vi "Sleep.vi"(8 "error in (no error)":errorcluster, 11 "ISleepableBaby in":refnum<class "ISleepableBaby.lvclass">) -> (0 "error out":errorcluster, 3 "ISleepableBaby out":refnum<class "ISleepableBaby.lvclass">)   [LabVIEW 2009, in "ISleepableBaby.lvclass"]
doc: "Cuddle with baby until she goes to sleep."
uses:
  ISleepableBaby.lvclass
  Baby.lvclass
  Source/IUnknown Class/IUnknown.lvclass
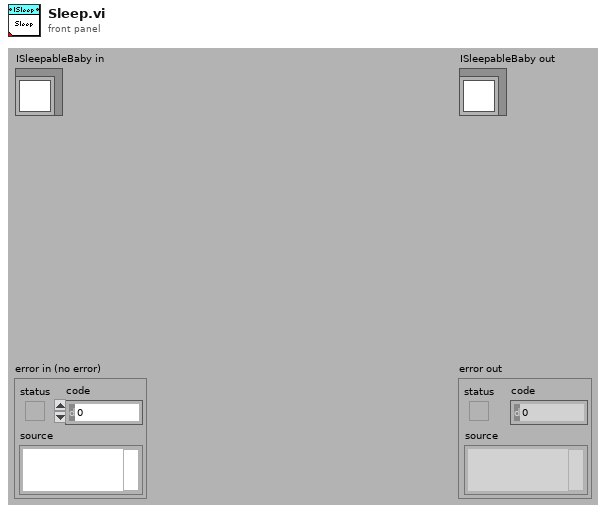
[diagram p1: front panel]
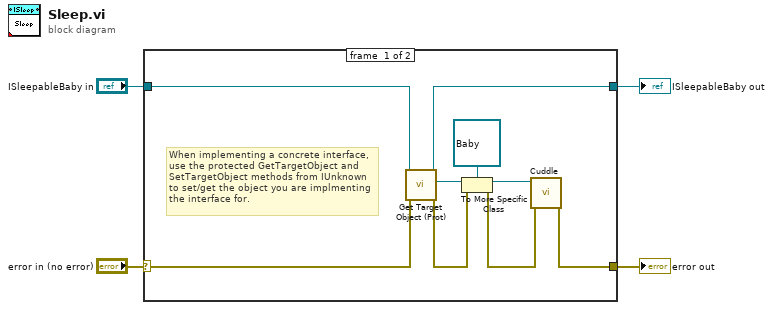
[diagram p0: block diagram]
diagram:
  n1 = case shown="No Error" "error in (no error)" {
    selector: "error in (no error)" -> [w5 w14]
    tunnel: "ISleepableBaby in" -> [w13 w15]
    tunnel: [w12 w15] -> w3
    tunnel: [w6 w14] -> w2
    frame #0 {
      # "When implementing a concrete interface,\nuse the protected GetTargetObject and SetTargetObject methods from IUnknown to set/get the object you are implmenting the interface for."
      n2 = call "Get Target Object (Prot).vi"("error in (no error)"=w5, "IUnknown in"=w13) -> ("error out"=w8:errorcluster, "Target Object"=w9:refnum<class "Interfaceable.lvclass">, "IUnknown out"=w12:refnum<class "ISleepableBaby.lvclass">)  [unwired: 7 in]
      n3 = To More Specific Class(target class=refnum<class "Baby.lvclass"> refnum ("Baby"), reference=w9, error in=w8) -> (specific class reference=w10:refnum<class "Baby.lvclass">, error out=w7:errorcluster)
      n4 = call "Cuddle.vi"("error in (no error)"=w7, "Baby in"=w10) -> ("error out"=w6:errorcluster)  [unwired: 8 in, 1 out]
    }
    frame #1 {
    }
  }
  "error out" <- w2
  "ISleepableBaby out" <- w3
